vi "Set current step.vi"(11 "Waveform parameters":T1 {"StartCurrent" min=0.001}) -> (3 "Waveform parameters out":T1={"StartCurrent"=1.0, "MaximumCurrent (mA)"=3.0, "Number oif pulses"=3, "Ramp length"=20, "Top length"=4, "Exponent"=1, "CurrentStep "=1.0, "Baseline length"=8, "Next current step"=0.0} {"StartCurrent" min=0.001})   [LabVIEW 2015]
uses:
  Original Waveform parameters.ctl
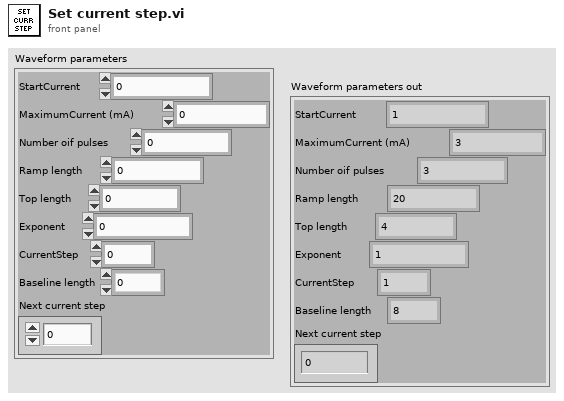
[diagram p1: front panel]
types:
  T1 = typedef "Original Waveform parameters.ctl" = cluster{"StartCurrent":dbl, "MaximumCurrent (mA)":dbl, "Number oif pulses":i32, "Ramp length":i32, "Top length":i32, "Exponent":i16, "CurrentStep ":dbl, "Baseline length":i32, "Next current step":dbl}
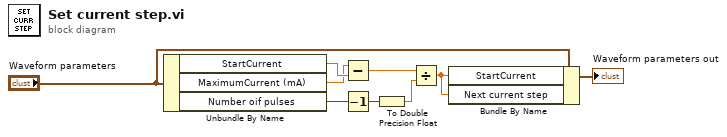
[diagram p0: block diagram]
diagram:
  n1 = Unbundle By Name("Waveform parameters") -> ("StartCurrent"=w5:dbl, "MaximumCurrent (mA)"=w4:dbl, "Number oif pulses"=w7:i32)
  n2 = Subtract(x=w4, y=w5) -> (x-y=w6:dbl)
  n3 = Decrement(x=w7) -> (x-1=w8:i32)
  n4 = To Double Precision Float(number=w8) -> (double precision float=w9:dbl)
  n5 = Divide(x=w6, y=w9) -> (x/y=w1:dbl)
  n6 = Bundle By Name(cluster="Waveform parameters", "StartCurrent"=w1, "Next current step"=w1) -> (→"Waveform parameters out":T1)
